vi "FXP-I32 Conversion test.vi"() -> ()   [LabVIEW 2018]
panel:
  out "Waveform Graph 2":i32[](graph)
  out "Output 2":i32
  out "Waveform Graph":i32[](graph)
  out "Output":i32
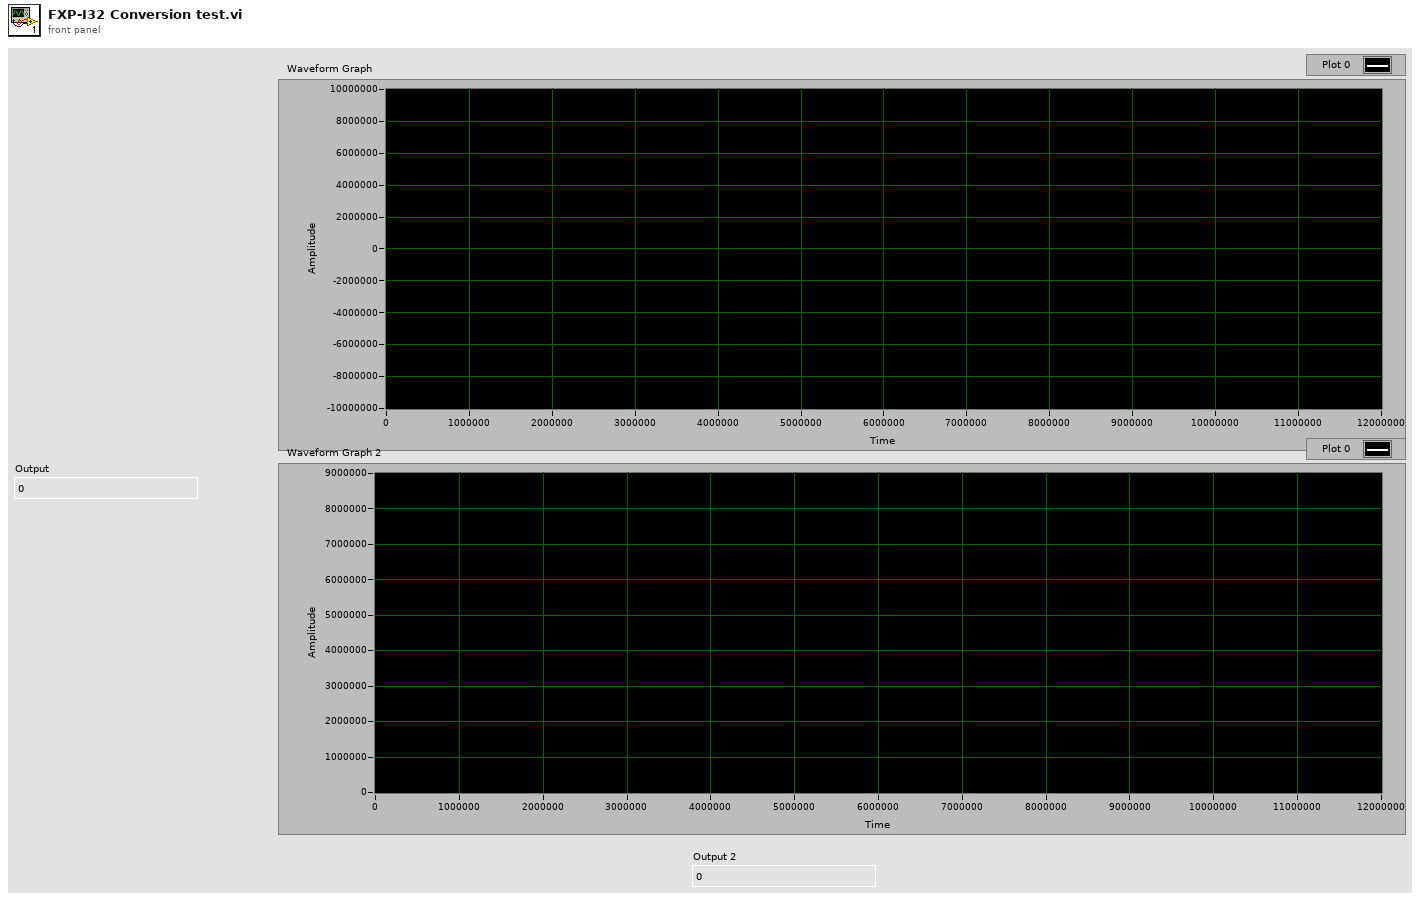
[diagram p1: front panel]
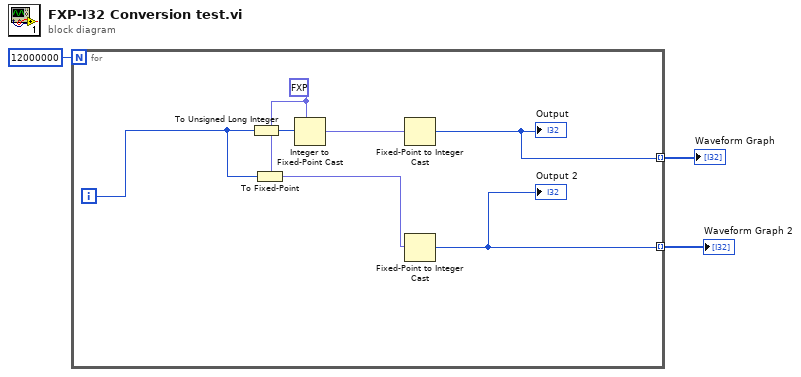
[diagram p0: block diagram]
diagram:
  n1 = for {
    N: 12000000 -> [_]
    tunnel: [w8] -> w3 mode=indexing
    tunnel: [w5] -> w1 mode=indexing
    i -> [w7]
    w4 = fxp<+/-,24,1> 0.0 ("fixed-point type")
    n2 = To Unsigned Long Integer(number=w7) -> (unsigned 32bit integer=w9:u32)
    n3 = To Fixed-Point(fixed-point type=w4, number=w7) -> (fixed-point=w6:fxp<+/-,24,1>)
    n4 = Integer to Fixed-Point Cast(fixed-point type=w4, integer=w9) -> (fixed-point=w10:fxp<+/-,24,1>)
    n5 = Fixed-Point to Integer Cast(1:w10) -> (0:w8:i32)
    "Output" <- w8
    n6 = Fixed-Point to Integer Cast(1:w6) -> (0:w5:i32)
    "Output 2" <- w5
  }
  "Waveform Graph" <- w3
  "Waveform Graph 2" <- w1
